vi "Memory.Pointer.Write.Safe.1D.I8.vi"(8 "error in (no error)":errorcluster, 9 "count":u64 format="%d elements", 10 "buffer in":i8[](array[numeric]), 11 "pointer in":refnum<class "Memory.Pointer.lvclass">) -> (0 "error out":errorcluster, 2 "buffer out":i8[](array[numeric]), 3 "pointer out":refnum<class "Memory.Pointer.lvclass">)   [LabVIEW 2016, in "Memory Manager.lvlib" / "Memory.Pointer.lvclass"]
doc: "Writes <b>count</b> elements from the provided <b>buffer</b> to the address specified by <b>pointer</b>.\n\n<b>Note:</b> This VI is <b>safe</b>.\n\nSafe means that this function evaluates the size parameter of <b>pointer</b> to ensure that is inbounds of allocated memory before peforming a memory read/write. Reading/writing more data to a pointer than it has allocated can corrupt or crash LabVIEW."
uses:
  Memory.Pointer.lvclass
  Memory.Pointer.lvclass/Memory.Pointer.ctl
  Accessors/Get Address.vi
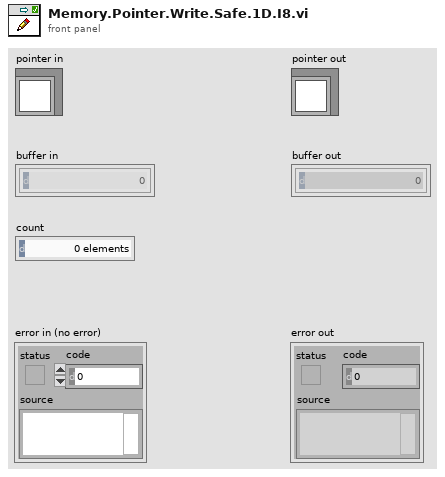
[diagram p1: front panel]
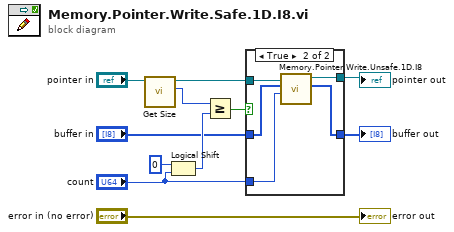
[diagram p0: block diagram]
diagram:
  n1 = call "Get Size.vi"("Pointer in"="pointer in") -> ("size"=w9:u64, "Pointer out"=w6:refnum<class "Memory.Pointer.lvclass">)  [unwired: 8 in, 1 out]
  n2 = Logical Shift(y=i16 0, x="count") -> (x << y=w7:u64)
  n3 = Greater Or Equal?(x=w9, y=w7) -> (x >= y?=w2:bool)
  n4 = case shown="True" w2 {
    tunnel: "count" -> [_ w15]
    tunnel: w6 -> [w12 w18]
    tunnel: [w12 w17] -> w5
    tunnel: "buffer in" -> [w13 w16]
    tunnel: [w13 w14] -> w3
    frame False {
    }
    frame True {
      n5 = call "Memory.Pointer.Write.Unsafe.1D.I8.vi"("count"=w15, "buffer in"=w16, "pointer in"=w18) -> ("buffer out"=w14:i8[], "pointer out"=w17:refnum<class "Memory.Pointer.lvclass">)  [unwired: 6 in, 1 out]
    }
  }
  "pointer out" <- w5
  "buffer out" <- w3
  "error out" <- "error in (no error)"
